vi "Read_SG_JPG.vi"(4 "Plane":i32 min=0 step=1, 6 "Scale cluster":cluster{"Start":dbl, "scale":dbl}={"Start"=0.0, "scale"=1.0}, 7 "B1 Set":bool, 8 "Divider":i32[](array[numeric])=[10, 5], 9 "Array Dims":i32[](array[numeric]), 10 "in coordinates":T1, 11 "directory path":path) -> (2 "SG":picture, 3 "concatenated string":string)   [LabVIEW 2022 SP3]
uses:
  <vilib>/Utility/miscctls.llb/LVPointDoubleTypeDef.ctl
  <vilib>/Utility/file.llb/Read Delimited Spreadsheet (DBL).vi
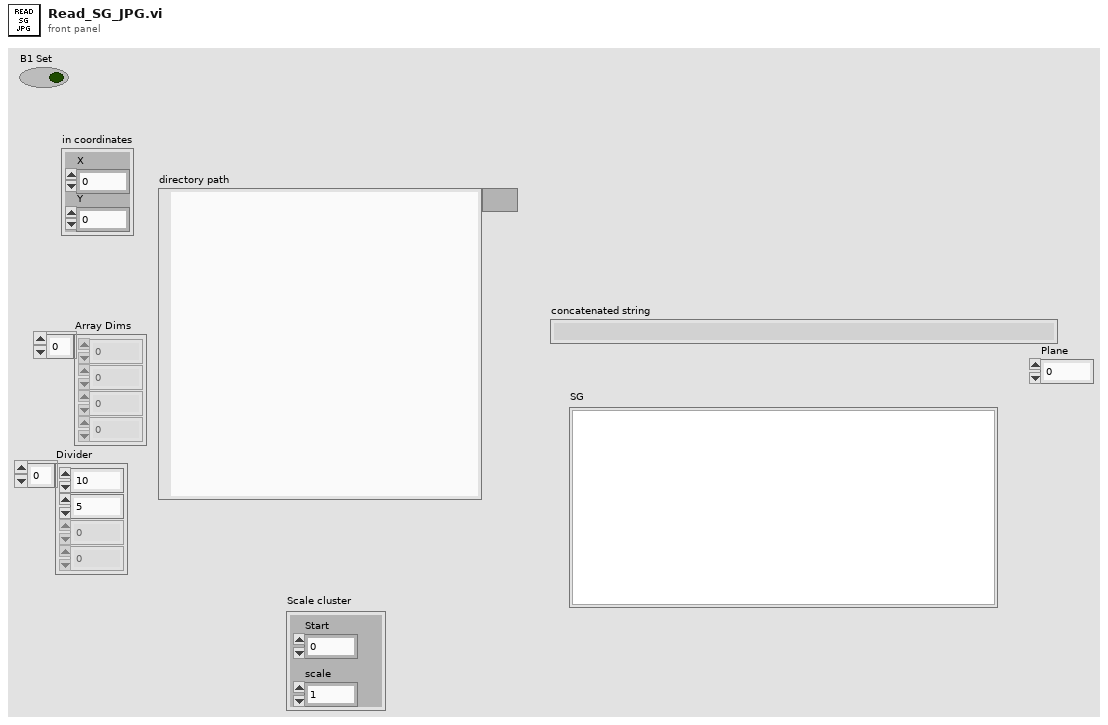
[diagram p1: front panel]
types:
  T1 = typedef "LVPointDoubleTypeDef.ctl" = cluster{"X":dbl, "Y":dbl}
  T2 = cluster{"left":i16, "top":i16, "right":i16, "bottom":i16}
  T3 = typedef "imagedata.ctl" = cluster{"image type":i32, "image depth":i32, "image":u8[], "mask":u8[], "colors":u32[], "Rectangle":cluster{"left":i16, "top":i16, "right":i16, "bottom":i16}}
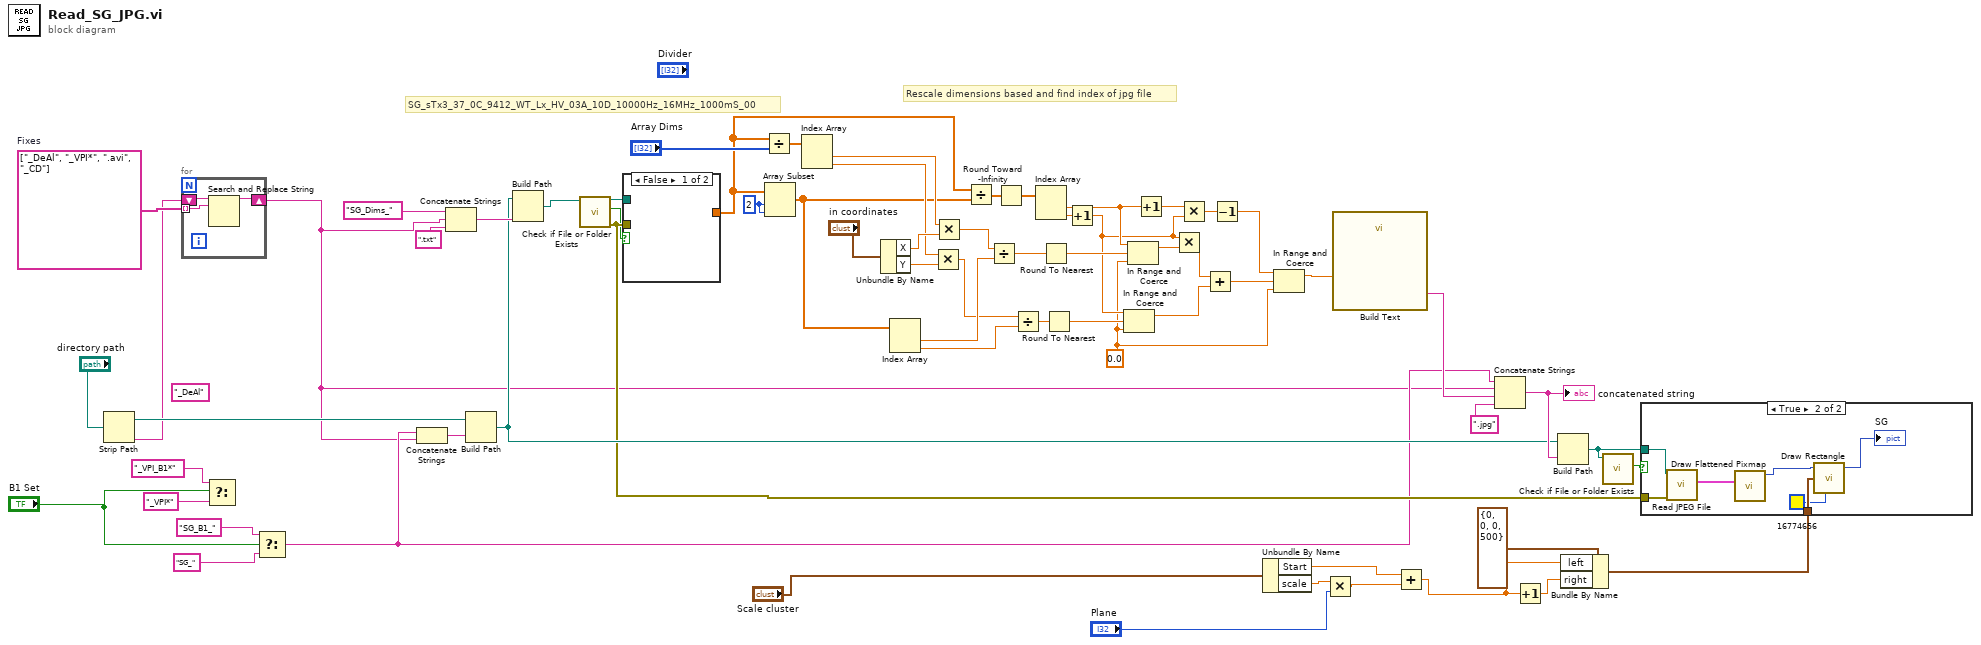
[diagram p0: block diagram]
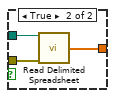
[diagram p2: hidden frame]
diagram:
  w3 = string[] ["_DeAl", "_VPI*", ".avi", "_CD"]  # Fixes
  (unwired) "_DeAl" ("search string")
  w34 = 2 ("index")
  w28 = 0.0 ("lower limit")
  # "SG_sTx3_37_0C_9412_WT_Lx_HV_03A_10D_10000Hz_16MHz_1000mS_00"
  # "Rescale dimensions based and find index of jpg file"
  n1 = Strip Path(path="directory path") -> (stripped path=w61:path, name=w2:string)
  n2 = for {
    tunnel: w3 -> [w68] mode=indexing
    shift-right: [w67] -> w1
    shift-left: w2 -> [w69]
    n3 = Search and Replace String(input string=w69, search string=w68) -> (result string=w67:string)  [unwired: 6 in, 3 out]
  }
  n4 = Select(t="_VPI_B1*" ("search string"), s="B1 Set", f="_VPI*" ("search string")) -> ()  [unwired: 1 out]
  n5 = Select(t="SG_B1_" ("string"), s="B1 Set", f="SG_" ("string")) -> (s? t:f=w14:string)
  n6 = Concatenate Strings(w14, w1) -> (w64:string)
  n7 = Concatenate Strings("SG_Dims_" ("string"), w1, ".txt" ("string")) -> (w45:string)
  n8 = Build Path(base path=w61, name or relative path=w64) -> (appended path=w44:path)
  n9 = Build Path(base path=w44, name or relative path=w45) -> (appended path=w24:path)
  n10 = call <vilib>:"Check if File or Folder Exists.vi"("path"=w24) -> ("error out"=w23:errorcluster, "file or folder exists?"=w21:bool, "dup path"=w22:path)  [unwired: 8 in]
  n11 = case shown="False" w21 {
    tunnel: [_ w72] -> w35
    tunnel: w23 -> [_ w71]
    tunnel: w22 -> [_ w70]
    frame False {
    }
    frame True {
      n12 = call-poly <vilib>:"Read Delimited Spreadsheet.vi"("file path (dialog if empty)"=w70, "error in (no error)"=w71) -> ("first row"=w72:dbl[])  [unwired: 8 in, 5 out]
    }
  }
  n13 = Divide(x=w35, y="Array Dims") -> (x/y=w42:dbl[])
  n14 = Array Subset(array=w35, index=w34, length=w34) -> (w33:dbl[])
  n15 = Index Array(array=w42) -> (element #1=w40:dbl, element #2=w37:dbl)  [unwired: 2 in]
  n16 = Unbundle By Name("in coordinates") -> ("X"=w41:dbl, "Y"=w38:dbl)
  n17 = Index Array(array=w33) -> (element #1=w54:dbl, element #2=w53:dbl)  [unwired: 2 in]
  n18 = Multiply(x=w37, y=w38) -> (x*y=w36:dbl)
  n19 = Multiply(x=w40, y=w41) -> (x*y=w39:dbl)
  n20 = Divide(x=w35, y=w33) -> (x/y=w59:dbl[])
  n21 = Divide(x=w39, y=w54) -> (x/y=w55:dbl)
  n22 = Round Toward -Infinity(1:w59) -> (0:w58:dbl[])
  n23 = Divide(x=w36, y=w53) -> (x/y=w65:dbl)
  n24 = Index Array(array=w58) -> (element #1=w32:dbl, element #2=w48:dbl)  [unwired: 2 in]
  n25 = Round To Nearest(number=w55) -> (nearest integer value=w50:dbl)
  n26 = Round To Nearest(number=w65) -> (nearest integer value=w52:dbl)
  n27 = Increment(x=w48) -> (x+1=w31:dbl)
  n28 = In Range and Coerce(upper limit=w31, x=w52, lower limit=w28) -> (coerced(x)=w51:dbl)  [unwired: 1 out]
  n29 = In Range and Coerce(upper limit=w32, x=w50, lower limit=w28) -> (coerced(x)=w49:dbl)  [unwired: 1 out]
  n30 = Increment(x=w32) -> (x+1=w25:dbl)
  n31 = Multiply(x=w31, y=w49) -> (x*y=w57:dbl)
  n32 = Multiply(x=w25, y=w31) -> (x*y=w29:dbl)
  n33 = Add(x=w57, y=w51) -> (x+y=w30:dbl)
  n34 = Decrement(x=w29) -> (x-1=w26:dbl)
  n35 = Unbundle By Name("Scale cluster") -> ("Start"=w9:dbl, "scale"=w10:dbl)
  n36 = In Range and Coerce(upper limit=w26, x=w30, lower limit=w28) -> (coerced(x)=w27:dbl)  [unwired: 1 out]
  n37 = Multiply(x=w10, y="Plane") -> (x*y=w4:dbl)
  n38 = call "Build Text"("name"=w27) -> ("Result"=w63:string)  [unwired: 13 in, 1 out]
  n39 = Add(x=w9, y=w4) -> (x+y=w7:dbl)
  n40 = Concatenate Strings(w14, w1, w63, ".jpg" ("string")) -> (w62:string)
  "concatenated string" <- w62
  n41 = Increment(x=w7) -> (x+1=w5:dbl)
  n42 = Build Path(base path=w44, name or relative path=w62) -> (appended path=w20:path)
  n43 = Bundle By Name(cluster=T2 {"left"=0, "top"=0, "right"=0, "bottom"=500} ("rect"), "left"=w7, "right"=w5) -> (w6:T2)
  n44 = call <vilib>:"Check if File or Folder Exists.vi"("path"=w20) -> ("file or folder exists?"=w19:bool)  [unwired: 8 in, 2 out]
  n45 = case shown="True" w19 {
    tunnel: w20 -> [_ w79]
    tunnel: w23 -> [_ w77]
    tunnel: w6 -> [_ w74]
    frame False {
    }
    frame True {
      n46 = call <vilib>:"Read JPEG File.vi"("error in (no error)"=w77, "path to JPEG file"=w79) -> ("image data"=w78:T3)  [unwired: 7 in, 2 out]
      n47 = call <vilib>:"Draw Flattened Pixmap.vi"("image data"=w78) -> ("new picture"=w76:picture)  [unwired: 8 in]
      n48 = call <vilib>:"Draw Rectangle.vi"("picture"=w76, "rect"=w74, "color(black)"=u32 16774656) -> ("new picture"=→"SG":picture)  [unwired: 6 in]
    }
  }
